vi "InitMiscellaneous.vi"   [LabVIEW 2019]
doc: "This VI initializes miscellaneous devices such as the compressor and any decorations."
uses:
  <vilib>/Rock Robotics/SystemInterfaces/DIO/FPGA_DIOPWMChannel.ctl
  refnums.vi
  outputs.vi
  <vilib>/Rock Robotics/WPI/Utilities/WPI_GetSetVariantRefNum.vi
types:
  T1 = typedef "FPGA_DIOPWMChannel.ctl" = enum8{"PWM 0", "PWM 1", "PWM 2", "PWM 3", "PWM 4", "PWM 5", "PWM 6", "PWM 7", "PWM 8", "PWM 9", "PWM MXP 0", "PWM MXP 1", "PWM MXP 2", "PWM MXP 3", "PWM MXP 4", "PWM MXP 5", "PWM MXP 6", "PWM MXP 7", "PWM MXP 8", "PWM MXP 9", "Invalid"}
  T2 = typedef "WPI_CompressorDevRef.ctl" = cluster{"DevStatus":errorcluster, "Pneumatics Control Module":u8}
  T3 = typedef "WPI_PWMDeviceRef.ctl" = cluster{"DeviceStatus":errorcluster, "PWM Channel":T1}
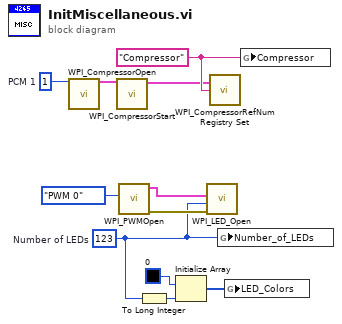
[diagram p0: block diagram]
diagram:
  w4 = "Compressor" ("refnum name")
  w2 = u8 1  # PCM 1
  w7 = u16 123  # Number of LEDs
  n1 = call <vilib>:"WPI_CompressorOpen.vi"("Pneumatics Control Module (0)"=w2) -> ("CompressorDevRef"=w1:T2)  [unwired: 13 in, 1 out]
  n2 = call <vilib>:"WPI_CompressorStart.vi"("CompressorDevRef"=w1) -> ("CompressorDevRef"=w3:T2)  [unwired: 9 in, 1 out]
  n3 = call <vilib>:"WPI_PWMOpen.vi"("PWM Channel"=FPGA_DIOPWMChannel."PWM 0") -> ("error out"=w10:errorcluster, "PWMDeviceRef"=w11:T3)  [unwired: 9 in]
  n4 = To Long Integer(number=w7) -> (32bit integer=w8:i32)
  n5 = Initialize Array(u32 0, w8) -> (w5:u32[])
  n6 = call <vilib>:"WPI_LED_Open.vi"("error in"=w10, "String Length"=w7, "PWMDeviceRef"=w11) -> ()  [unwired: 8 in, 1 out]
  n7 = call <vilib>:"WPI_CompressorRefNum Registry Set.vi"("refnum name"=w4, "CompressorDevRef"=w3) -> ()  [unwired: 8 in, 2 out]
  n8 = global write "refnums.vi" "Number_of_LEDs"(w7) -> ()
  n9 = global write "outputs.vi" "LED_Colors"(w5) -> ()
  n10 = global write "refnums.vi" "Compressor"(w4) -> ()
